vi "freqToStringvi.vi"(8 "error in (no error)":errorcluster, 11 "SingleTone in":refnum<class "SingleTone.lvclass">) -> (0 "error out":errorcluster, 2 "frequency":string, 3 "SingleTone out":refnum<class "SingleTone.lvclass">)   [LabVIEW 2011, in "Tools.lvlib" / "Scripting.lvlib" / "SingleTone.lvclass"]
uses:
  SingleTone.lvclass
  SingleTone.lvclass/SingleTone.ctl
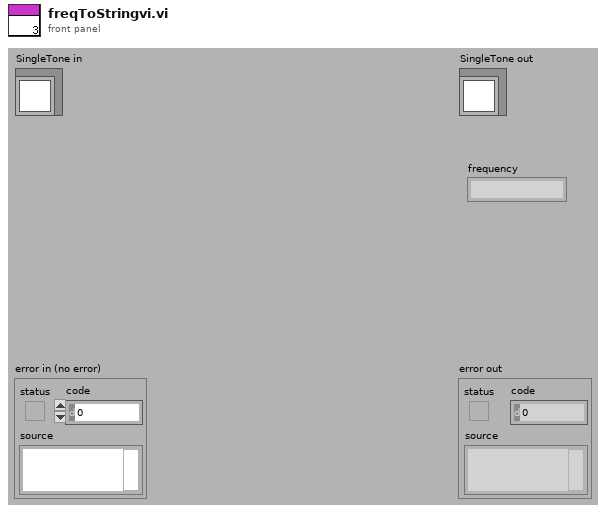
[diagram p1: front panel]
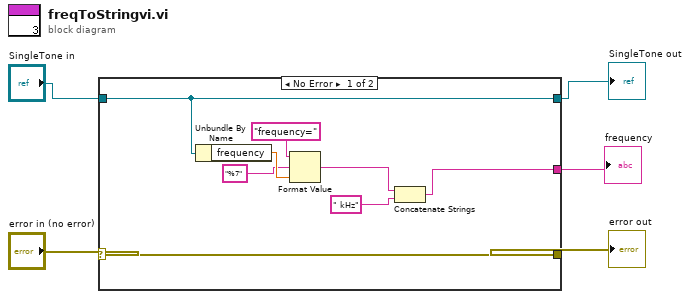
[diagram p0: block diagram]
diagram:
  n1 = case shown="No Error" "error in (no error)" {
    selector: "error in (no error)" -> [w11 w14]
    tunnel: [w11 w14] -> w4
    tunnel: [w10 w15] -> w2
    tunnel: "SingleTone in" -> [w10 w15]
    tunnel: [w6 _] -> w1
    frame No Error {
      n2 = Unbundle By Name(w10) -> ("frequency"=w13:dbl)
      n3 = Format Value(string ("")="frequency=", format string="%7", value (0)=w13) -> (output string=w7:string)
      n4 = Concatenate Strings(w7, " kHz") -> (w6:string)
    }
    frame Error {
    }
  }
  "error out" <- w4
  "SingleTone out" <- w2
  "frequency" <- w1
